vi "AttackerBallOutOfFieldTactic.vi"(8 "error in (no error)":errorcluster, 9 "Game in":refnum<class "Game.lvclass">, 10 "Robot":refnum<class "Robot.lvclass">, 11 "AttackerBallOutOfFieldTactic in":refnum<class "AttackerBallOutOfFieldTactic.lvclass">) -> (0 "error out":errorcluster, 2 "Robot out":refnum<class "Robot.lvclass">, 3 "AttackerBallOutOfFieldTactic out":refnum<class "AttackerBallOutOfFieldTactic.lvclass">)   [LabVIEW 2018, in "AttackerBallOutOfFieldTactic.lvclass"]
uses:
  AttackerBallOutOfFieldTactic.lvclass
  C:/Users/Gustavo/Desktop/RoboIME/SimplePass/SSL_AI/Tactic_class/Tactic.lvclass
  Robot_class/Robot.lvclass
  Game_class/Game.lvclass
  Tactic_class/Tactic.lvclass/Tactic.ctl
  States.ctl
  Robot_class/tactics.ctl
  Skillbook_class/Skillbook.lvclass/Skillbook.ctl
  Game_class/Game.lvclass/Game.ctl
  Parameters_class/Parameters.lvclass/Parameters.ctl
  AttackerBallOutOfFieldTactic.lvclass/AttackerBallOutOfFieldTactic.ctl
  Robot_class/Robot.lvclass/Robot.ctl
  Game_class/Read Parameters.lvclass.vi
  Parameters_class/Read DistanceToBallOut.vi
  Skillbook_class/Read AttackerBallOutOfFieldSkill.vi
  Tactic_class/Read Skillbook.vi
  Robot_class/Write tactic.vi
  Write States.vi
  Skillbook_class/Skillbook.lvclass
  Parameters_class/Parameters.lvclass
  AttackerBallOutOfFieldSkill_class/AttackerBallOutOfFieldSkill.lvclass
panel:
  out "x .or. y?":bool
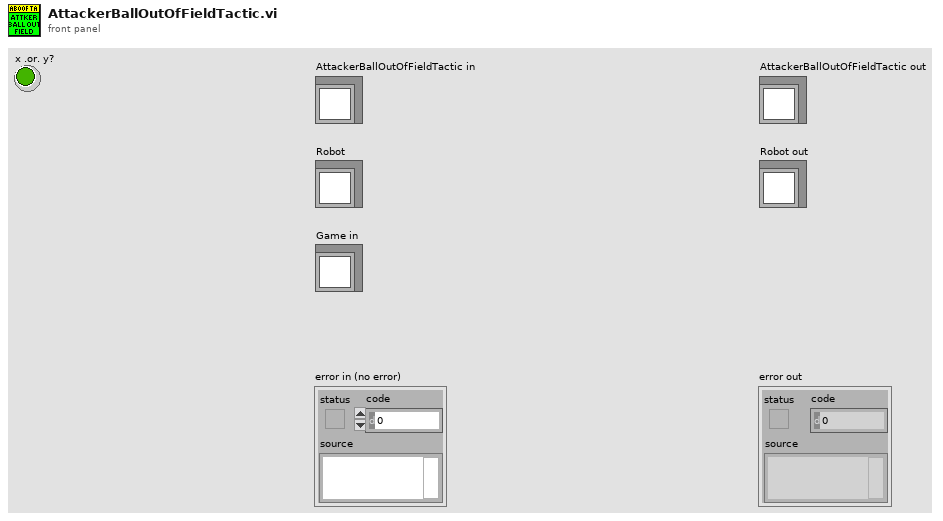
[diagram p1: front panel]
types:
  T1 = typedef "tactics.ctl" = enum16{"PenaltyAttacker", "PassObserver", "PenaltyDefense", "Test", "DefendGoal", "Marker", "FollowAttacker", "DefendArea", "Shoot", "AttackerAimGoal", "AttackerBallOutOfField", "AttackerBlock", "AttackerStop", "Duelist", "Halt", "ZigZag", "GoTo", "Timeout", "KickToPassReceiver", "PositionToReceivePass", "PassReceiver", "WaitPass"}
  T2 = typedef "AttackerBallOutOfFieldTactic.lvclass/States.ctl" = enum16{"Exit", "BallOutOfField"}
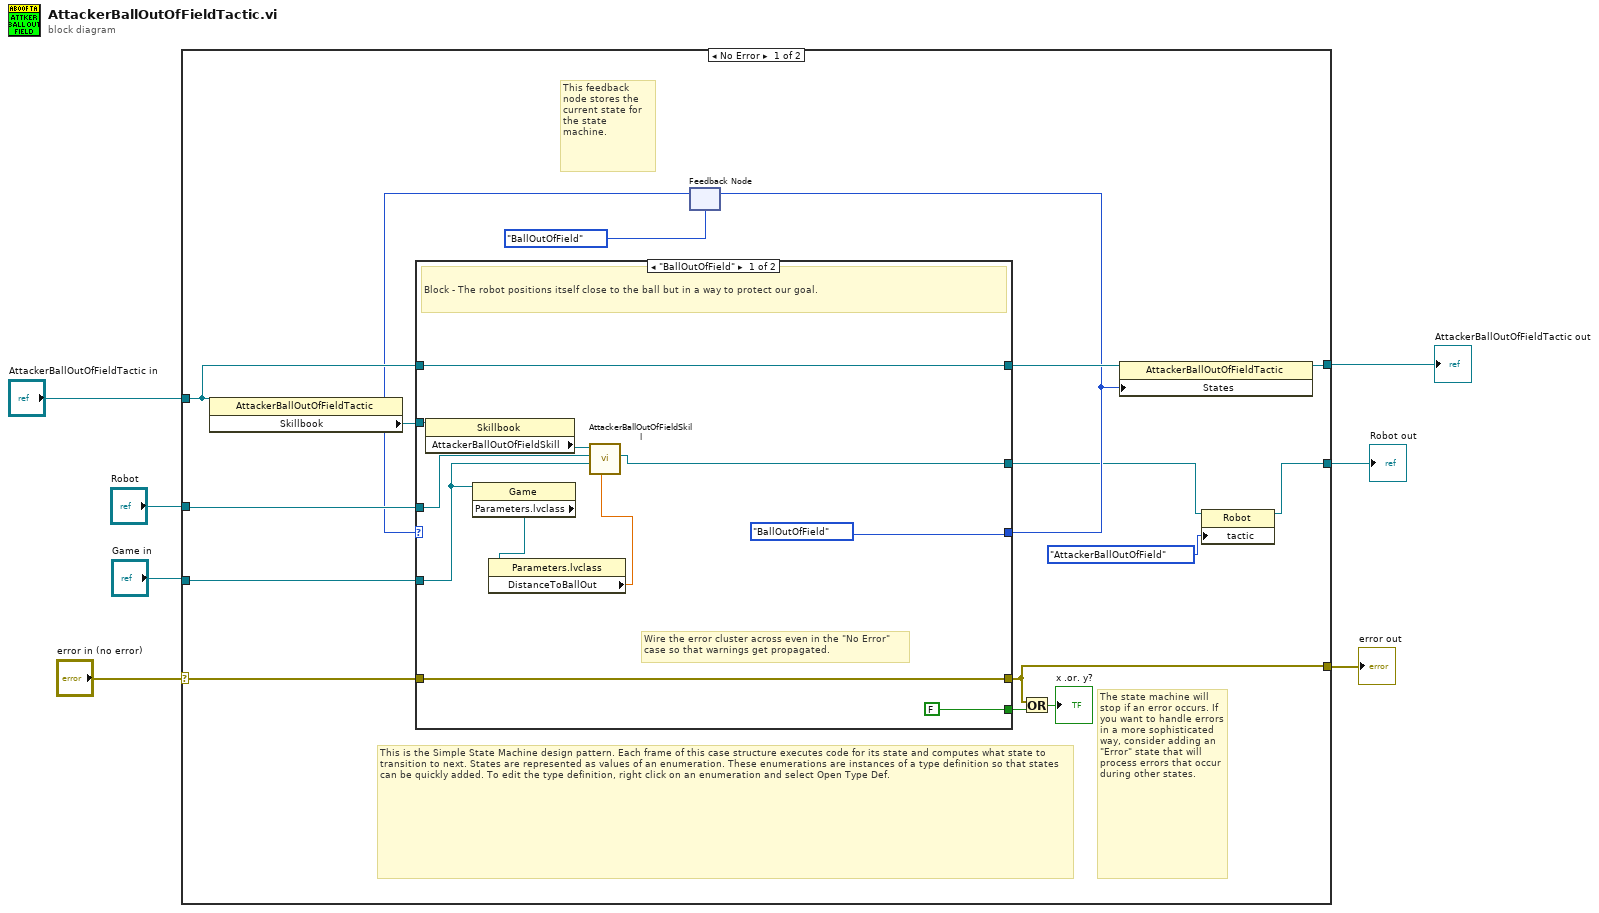
[diagram p0: block diagram]
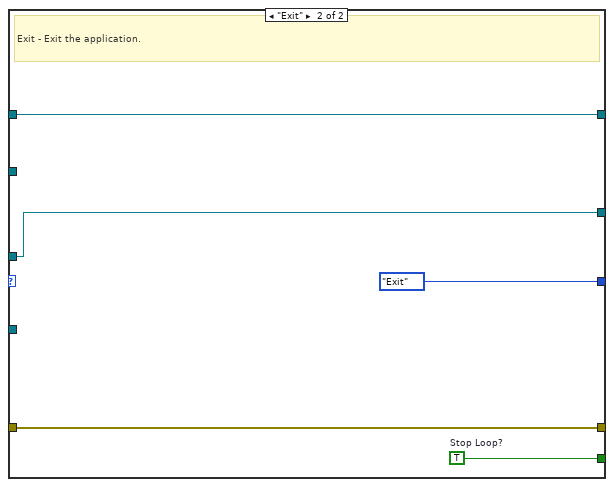
[diagram p2: hidden frame]
diagram:
  n1 = case shown="No Error" "error in (no error)" {
    selector: "error in (no error)" -> [w16 w42]
    tunnel: [w15 w42] -> w6
    tunnel: [w11 w41] -> w5
    tunnel: "Robot" -> [w18 w40]
    tunnel: "Game in" -> [w17 _]
    tunnel: "AttackerBallOutOfFieldTactic in" -> [w14 w41]
    tunnel: [w8 w40] -> w1
    frame No Error {
      # "The state machine will stop if an error occurs. If you want to handle errors in a more sophisticated way, consider adding an \"Error\" state that will process errors that occur during other states."
      # "This feedback node stores the current state for the state machine."
      # "This is the Simple State Machine design pattern. Each frame of this case structure executes code for its state and computes what state to transition to next. States are represented as values of an enumeration. These enumerations are instances of a type definition so that states can be quickly added. To edit the type definition, right click on an enumeration and select Open Type Def."
      # "Wire the error cluster across even in the \"No Error\"\ncase so that warnings get propagated."
      n2 = property class="AttackerBallOutOfFieldTactic"(reference=w14) -> ("Skillbook"=w21:refnum<class "Skillbook.lvclass">)  [unwired: 1 in, 2 out]
      n3 = feedback #1(States."BallOutOfField" ("States")) -> (w12:T2)
      n4 = case shown="\"BallOutOfField\"" w12 {
        tunnel: [States."BallOutOfField" ("States") States."Exit" ("States")] -> w19
        tunnel: [FALSE ("Stop Loop?") w39] -> w23
        tunnel: w16 -> [w33 w38]
        tunnel: [w33 w38] -> w15
        tunnel: w21 -> [w32 _]
        tunnel: w18 -> [w26 w37]
        tunnel: [w24 w37] -> w9
        tunnel: [w31 w36] -> w20
        tunnel: w14 -> [w31 w36]
        tunnel: w17 -> [w29 _]
        frame "BallOutOfField" {
          # "Block - The robot positions itself close to the ball but in a way to protect our goal."
          n5 = property class="Skillbook"(reference=w32) -> ("AttackerBallOutOfFieldSkill"=w30:refnum<class "AttackerBallOutOfFieldSkill.lvclass">)  [unwired: 1 in, 2 out]
          n6 = property class="Game"(reference=w29) -> ("Parameters.lvclass"=w28:refnum<class "Parameters.lvclass">)  [unwired: 1 in, 2 out]
          n7 = property class="Parameters.lvclass"(reference=w28) -> ("DistanceToBallOut"=w27:dbl)  [unwired: 1 in, 2 out]
          n8 = call-dynamic "AttackerBallOutOfFieldSkill.vi"("DistanceToBallOut"=w27, "Game"=w29, "Robot"=w26, "AttackerBallOutOfFieldSkill in"=w30) -> ("Robot out"=w24:refnum<class "Robot.lvclass">)  [unwired: 5 in, 2 out]
        }
        frame "Exit" {
          w39 = TRUE  # Stop Loop?
          # "Exit - Exit the application."
        }
      }
      n9 = feedback-in #1(w19) -> ()
      n10 = Or(x=w15, y=w23) -> (x .or. y?=→"x .or. y?":bool)
      n11 = property class="AttackerBallOutOfFieldTactic"(reference=w20, "States"=w19) -> (reference out=w11:refnum<class "AttackerBallOutOfFieldTactic.lvclass">)  [unwired: 1 in, 1 out]
      n12 = property class="Robot"(reference=w9, "tactic"=tactics."AttackerBallOutOfField") -> (reference out=w8:refnum<class "Robot.lvclass">)  [unwired: 1 in, 1 out]
    }
    frame Error {
    }
  }
  "error out" <- w6
  "AttackerBallOutOfFieldTactic out" <- w5
  "Robot out" <- w1
